vi "PH_Cont-601k_PSU.ProcPeriodic.vi"(0 "i ref in":refnum<vi>, 3 "ms timeout (10000)":i32=10000, 5 "error in (no error)":errorcluster) -> (14 "i ref out":refnum<vi>, 17 "timed out":bool, 19 "error out":errorcluster)   [LabVIEW 2014, in "PH_Cont-601k_PSU.lvlib"]
doc: "This method serves to periodically do things like reading values from the HW. Methods that should be executed periodically should be called from THIS methode. Add code here."
uses:
  PH_Cont-601k_PSU.lvlib
  CSCore/CSSystem/CSSystemLib/CSSystemLib.lvlib
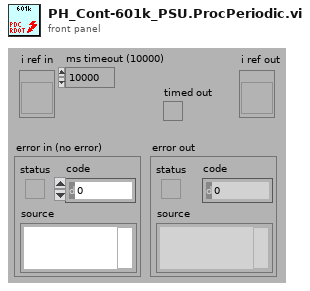
[diagram p1: front panel]
types:
  T1 = typedef "PH_Cont-601k_PSU.lvlib/PH_Cont-601k_PSU.i attribute.ctl" = cluster{"GUI Refs":T2, "Interlock":bool, "Service ID applied Voltage":i32, "Device Settings":cluster{"Configuration":T3, "Flash Interval [s]":dbl, "Mode":T4, "Voltage [V]":u16, "Charge":bool, "VISA resource name":refnum<visa-resource-name>}, "Readyness":T5, "Information":cluster{"VISA resource name":refnum<visa-resource-name>, "Tagname Power On":string, "Interlock":cluster{"Instance":string, "Tagname":string}, "Limits [V]":cluster{"Lower":dbl, "Upper":dbl}, "Tagname PSU On":string}, "R2S":bool, "Charge is allowed":bool}
  T2 = typedef "PH_Cont-601k_PSU.lvlib/PH_Cont-601k_PSU.GUI Refs.ctl" = cluster{"Power On":refnum<vi>, "Hard- and Software":refnum<vi>, "Device Status":refnum<vi>, "Device Error":refnum<vi>, "Configuration":refnum<vi>, "Flash Interval [s]":refnum<vi>, "Interlock":refnum<vi>, "Interlock Indicator":refnum<vi>, "Voltage [V]":refnum<vi>, "Readyness":refnum<vi>, "Mode":refnum<vi>, "Reset Error":refnum<vi>, "Expert working":refnum<vi>, "Charge":refnum<vi>, "PSU On":refnum<vi>}
  T3 = typedef "PH_Cont-601k_PSU.lvlib/PH_Cont-601k_PSU.Configuration.ctl" = u16
  T4 = typedef "PH_Cont-601k_PSU.lvlib/PH_Cont-601k_PSU.Mode.ctl" = enum32{"STOP", "STANDBY", "READY", "EMISSION", "ERROR"}
  T5 = typedef "PH_Cont-601k_PSU.lvlib/PH_Cont-601k_PSU.Readyness.ctl" = cluster{"Program":T6, "Device":T7}
  T6 = typedef "PH_Cont-601k_PSU.lvlib/PH_Cont-601k_PSU.Readyness Program.ctl" = enum32{"OFF", "POWER", "INTERLOCK"}
  T7 = typedef "PH_Cont-601k_PSU.lvlib/PH_Cont-601k_PSU.Readyness Device.ctl" = enum32{"OFF", "CONNECTING", "CONNECTED", "OPERATING", "EOC", "ERROR"}
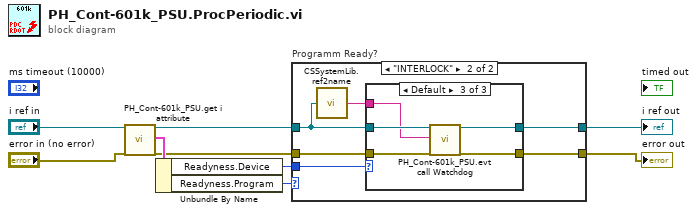
[diagram p0: block diagram]
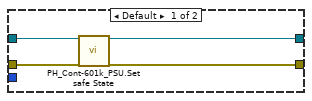
[diagram p2: hidden frame]
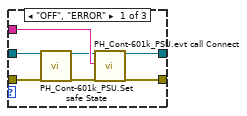
[diagram p3: hidden frame]
diagram:
  n1 = call "PH_Cont-601k_PSU.get i attribute.vi"("i ref in"="i ref in", "error in (no error)"="error in (no error)") -> ("i ref out"=w6:refnum<vi>, "i attribute"=w7:T1, "error out"=w5:errorcluster)  [unwired: 15 in]
  n2 = Unbundle By Name(w7) -> ("Readyness.Device"=w4:T7, "Readyness.Program"=w3:T6)
  n3 = case "Programm Ready?" shown="\"INTERLOCK\"" w3 {
    tunnel: w6 -> [w13 w15]
    tunnel: [w12 w17] -> w2
    tunnel: w5 -> [w11 w19]
    tunnel: [w10 w16] -> w1
    tunnel: w4 -> [_ w18]
    frame Default {
      n4 = call "PH_Cont-601k_PSU.Set safe State.vi"("VI in"=w13, "error in (no error)"=w11) -> ("VI out"=w12:refnum<vi>, "error out"=w10:errorcluster)  [unwired: 16 in]
    }
    frame "INTERLOCK" {
      n5 = call "CSSystemLib.ref2name.vi"("obj refnum"=w15) -> ("name"=w14:string)
      n6 = case shown="Default" w18 {
        tunnel: w15 -> [w23 w28 w33]
        tunnel: [w26 w28 w32] -> w17
        tunnel: w19 -> [w21 w27 w30]
        tunnel: [w25 w27 w29] -> w16
        tunnel: w14 -> [w24 _ w31]
        frame "OFF", "ERROR" {
          n7 = call "PH_Cont-601k_PSU.Set safe State.vi"("VI in"=w23, "error in (no error)"=w21) -> ("VI out"=w22:refnum<vi>, "error out"=w20:errorcluster)  [unwired: 16 in]
          n8 = call "PH_Cont-601k_PSU.evt call Connect.vi"("i ref in"=w22, "Instance"=w24, "error in (no error)"=w20) -> ("i ref out"=w26:refnum<vi>, "error out"=w25:errorcluster)  [unwired: 15 in]
        }
        frame "CONNECTING" {
        }
        frame Default {
          n9 = call "PH_Cont-601k_PSU.evt call Watchdog.vi"("i ref in"=w33, "Instance"=w31, "error in (no error)"=w30) -> ("i ref out"=w32:refnum<vi>, "error out"=w29:errorcluster)  [unwired: 15 in]
        }
      }
    }
  }
  "error out" <- w1
  "i ref out" <- w2
